vi "DFD FXP Simulation with State (I32).vi"(5 "input range":dbl=1.0, 6 "state in":dbl[](array[numeric]) format="%.2f", 8 "error in (no error)":errorcluster, 9 "filtering statistics in":T3(array[cluster])=[{"quantizer source"=0, "statistical information"={"max value"=-inf, "min value"=inf, "#overflows"=0, "#underflows"=0, "#operations"=0}}, {"quantizer source"=1, "statistical information"={"max value"=-inf, "min value"=inf, "#overflows"=0, "#underflows"=0, "#operations"=0}}, {"quantizer source"=2, "statistical information"={"max value"=-inf, "min value"=inf, "#overflows"=0, "#underflows"=0, "#operations"=0}}, {"quantizer source"=3, "statistical information"={"max value"=-inf, "min value"=inf, "#overflows"=0, "#underflows"=0, "#operations"=0}}, {"quantizer source"=4, "statistical information"={"max value"=-inf, "min value"=inf, "#overflows"=0, "#underflows"=0, "#operations"=0}}, {"quantizer source"=5, "statistical information"={"max value"=-inf, "min value"=inf, "#overflows"=0, "#underflows"=0, "#operations"=0}}, {"quantizer source"=6, "statistical information"={"max value"=-inf, "min value"=inf, "#overflows"=0, "#underflows"=0, "#operations"=0}}] {"statistical information"."min value" format="%.2f"; "statistical information"."max value" format="%.2f"; "quantizer source" items=["Coefficients a/k"=0, "Coefficients b/v"=7, "Input"=1, "Output"=2, "Multiplicand"=3, "Product"=4, "Sum"=5, "Delay"=6]}, 10 "filter in":T4={"mSRate_Fs"=1.0, "mSRate_Version"="2.0", "mSRate_Comments"="", "mSRate_OrgCoef"={"type"=enum."Undefined", "gain"=1.0, "coef a (k)"=[], "coef b (v)"=[]}, "mSRate_CurCoef"={"type"=enum."Undefined", "gain"=1.0, "coef a (k)"=[], "coef b (v)"=[]}, "mSRate_Quantized?"=FALSE, "mSRate_QCoef"={"type"=enum."Undefined", "gain"=1.0, "coef a (k)"=[], "coef b (v)"=[]}, "mSRate_QSettings"=[], "mSRate_Order"=0, "mSRate_Scaling"={"mSRate_ScaleByPowerOf2?"=FALSE, "mSRate_ScaleType"=enum."No Norm"}} {"mSRate_QSettings"."source" items=["Coef a/k"=0, "Coef b/v"=7, "Input"=1, "Output"=2, "Multiplicand"=3, "Product"=4, "Sum"=5, "Delay"=6, "Gain"=8]}, 11 "signal in":i32[](array[numeric])) -> (0 "error out":errorcluster, 1 "filtering statistics report":T3(array[cluster]) {"statistical information"."min value" format="%.2f"; "statistical information"."max value" format="%.2f"; "quantizer source" items=["Coefficients a/k"=0, "Coefficients b/v"=7, "Input"=1, "Output"=2, "Multiplicand"=3, "Product"=4, "Sum"=5, "Delay"=6]}, 2 "integer signal out":i32[](array[numeric]), 3 "DBL signal out":dbl[](array[numeric]) format="%.2f", 4 "state out":dbl[](array[numeric]) format="%.2f")   [LabVIEW 2017, in "NI_DigFilterLicensed.lvlib"]
doc: "Simulates the filtering process with initial internal states and generates the filtering statistics report for a fixed-point filter. The data type you wire to the <B>signal in</B> input determines the polymorphic instance to use."
uses:
  <vilib>/addons/Digital Filter Design/NI_DigFilterLicensed.lvlib
  <vilib>/addons/Digital Filter Design/_Objects.llb/DFD Filter Obj.ctl
  <vilib>/addons/Digital Filter Design/_Objects.llb/DFD Filter Coef.ctl
  <vilib>/addons/Digital Filter Design/_Objects.llb/DFD Filter Structure Type Selector.ctl
  <vilib>/addons/Digital Filter Design/_Objects.llb/dfd_Internal Quantization Settings.ctl
  <vilib>/addons/Digital Filter Design/_Objects.llb/dfd_Internal Quantization Srcs.ctl
  <vilib>/addons/Digital Filter Design/_Objects.llb/DFD Coef Norm Type.ctl
  <vilib>/addons/Digital Filter Design/_Objects.llb/DFD Quantization Sources.ctl
  <vilib>/addons/Digital Filter Design/_Objects.llb/DFD FXP Statistics Data.ctl
  <vilib>/addons/Digital Filter Design/NI_DigFilter_FXP.lvlib
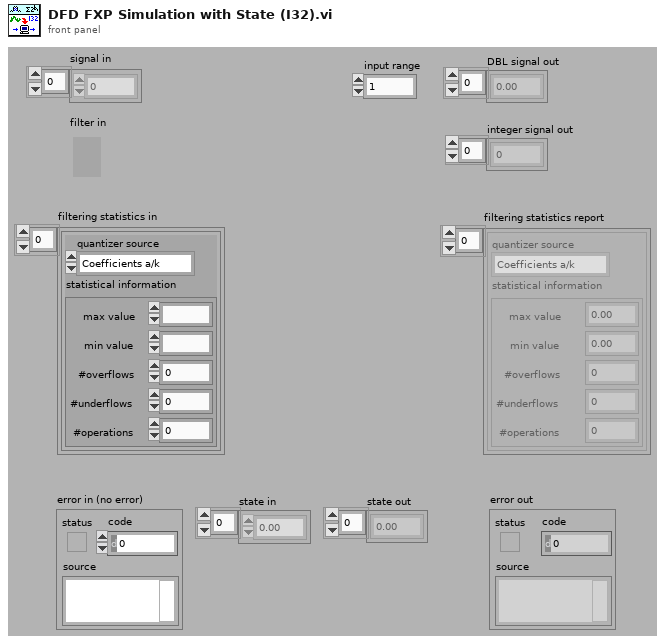
[diagram p1: front panel]
types:
  T1 = typedef "NI_DigFilterLicensed.lvlib/DFD Quantization Sources.ctl" = u16
  T2 = typedef "NI_DigFilterLicensed.lvlib/DFD FXP Statistics Data.ctl" = cluster{"max value":ext, "min value":ext, "#overflows":i32, "#underflows":i32, "#operations":i32}
  T3 = cluster{"quantizer source":T1, "statistical information":T2}[]
  T4 = typedef "NI_DigFilterLicensed.lvlib/DFD Filter Obj.ctl" = cluster{"mSRate_Fs":dbl, "mSRate_Version":string, "mSRate_Comments":string, "mSRate_OrgCoef":T5, "mSRate_CurCoef":T5, "mSRate_Quantized?":bool, "mSRate_QCoef":T5, "mSRate_QSettings":T7[], "mSRate_Order":i32, "mSRate_Scaling":cluster{"mSRate_ScaleByPowerOf2?":bool, "mSRate_ScaleType":T9}}
  T5 = typedef "NI_DigFilterLicensed.lvlib/DFD Filter Coef.ctl" = cluster{"type":T6, "gain":dbl, "coef a (k)":dbl[], "coef b (v)":dbl[]}
  T6 = typedef "NI_DigFilterLicensed.lvlib/DFD Filter Structure Type Selector.ctl" = enum16{"Undefined", "FIR Direct Form", "FIR Direct Form Transposed", "FIR Symmetric", "FIR Antisymmetric", "IIR Direct Form I", "IIR Direct Form I Transposed", "IIR Direct Form II", "IIR Direct Form II Transposed", "IIR Cascaded Second Order Sections Form I", "IIR Cascaded Second Order Sections Form I Transposed", "IIR Cascaded Second Order Sections Form II", "IIR Cascaded Second Order Sections Form II Transposed", "Lattice Allpass (basic sections)", "Lattice Allpass (one multiplier sections)", "Lattice Allpass (normalized sections)", "Lattice AR (basic sections)", "Lattice AR (one multiplier sections)", "Lattice AR (normalized sections)", "Lattice MA (minimum phase)", "Lattice MA (maximum phase)", "Lattice ARMA (basic sections)", "Lattice ARMA (one multiplier sections)", "Lattice ARMA (normalized sections)"}
  T7 = typedef "NI_DigFilterLicensed.lvlib/dfd_Internal Quantization Settings.ctl" = cluster{"source":T8, "wl":i16, "iwl":i16, "overflow mode":enum16{"Saturation", "Wrap"}, "rounding mode":enum16{"Nearest", "Truncation"}, "signed?":bool}
  T8 = typedef "NI_DigFilterLicensed.lvlib/dfd_Internal Quantization Srcs.ctl" = u16
  T9 = typedef "NI_DigFilterLicensed.lvlib/DFD Coef Norm Type.ctl" = enum16{"No Norm", "Time Domain 1-Norm", "Time Domain 2-Norm", "Time Domain Inf-Norm"}
  T10 = cluster{"Quantizer Source":T1, "statistics information":T2}[]
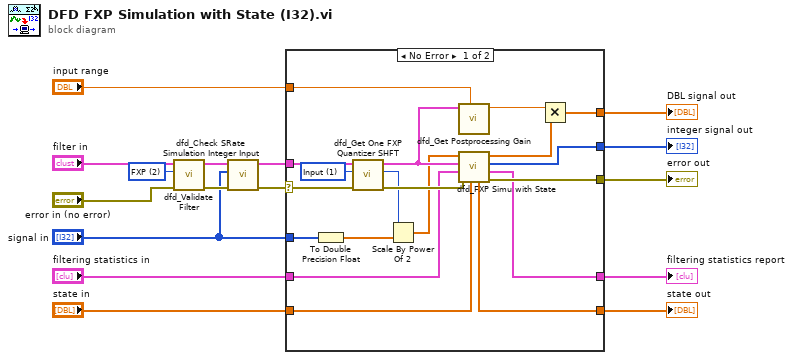
[diagram p0: block diagram]
diagram:
  w11 = u16 2 items=["Auto", "FLP Only", "FXP"] ("check option")
  n1 = call <vilib>:"dfd_Validate Filter.vi"("error in (no error)"="error in (no error)", "check option"=w11, "filter in"="filter in") -> ("error out"=w3:errorcluster, "filter out"=w12:T4)  [unwired: 7 out]
  n2 = call <vilib>:"dfd_Check SRate Simulation Integer Input.vi"("error in (no error)"=w3, "signal in"="signal in", "filter"=w12) -> ("error out"=w2:errorcluster, "dup multirate filter"=w4:T4)  [unwired: 7 out]
  n3 = case shown="No Error" w2 {
    selector: w2 -> [w33 w35]
    tunnel: "state in" -> [w26 _]
    tunnel: [w30 _] -> w15
    tunnel: [w34 w35] -> w14
    tunnel: [w27 _] -> w6
    tunnel: w4 -> [w24 _]
    tunnel: "input range" -> [w31 _]
    tunnel: "signal in" -> [w21 _]
    tunnel: "filtering statistics in" -> [w28 _]
    tunnel: [w25 _] -> w7
    tunnel: [w17 _] -> w5
    frame No Error {
      w22 = T8 1 items=["Coef a/k"=0, "Coef b/v"=7, "Input"=1, "Output"=2, "Multiplicand"=3, "Product"=4, "Sum"=5, "Delay"=6, "Gain"=8] ("quantization source")
      n4 = To Double Precision Float(number=w21) -> (double precision float=w20:dbl[])
      n5 = call <vilib>:"dfd_Get One FXP Quantizer SHFT.vi"("quantization source"=w22, "filter in"=w24) -> ("fwl SHFT"=w19:i16, "filter out"=w23:T4)  [unwired: 8 out]
      n6 = Scale By Power Of 2(n=w19, x=w20) -> (x*2^n=w18:dbl[])
      n7 = call <vilib>:"dfd_Get Postprocessing Gain.vi"("input range"=w31, "filter"=w23) -> ("integer gain"=w32:dbl)  [unwired: 9 out]
      n8 = call <vilib>:"dfd_FXP Simu with State.vi"("state in"=w26, "error in (no error)"=w33, "filtering statistics in"=w28, "filter"=w23, "signal in"=w18) -> ("error out"=w34:errorcluster, "filtering statistics out"=w27:T10, "integer signal out"=w17:i32[], "DBL signal out"=w29:dbl[], "state out"=w25:dbl[])  [unwired: 2 in]
      n9 = Multiply(x=w32, y=w29) -> (x*y=w30:dbl[])
    }
    frame Error {
    }
  }
  "DBL signal out" <- w15
  "error out" <- w14
  "state out" <- w7
  "filtering statistics report" <- w6
  "integer signal out" <- w5
